vi "Determine E-Series Level_2.vi"(3 "Number of Bands":u8=4 min=3 max=6 step=1, 5 "Tolerance (%)":dbl) -> (1 "E-Series Level":T1)   [LabVIEW 2018]
doc: "Determines the <b>E-Series Level</b> of a resistor based on its <b>Number of Bands</b> and <b>Tolerance (%)</b>.\n\nThe E-Series Level is an internal classification used by the application to determine which E-Series data must be evaluated for the resistor.\n\nThe classification is defined as follows:\n\nE-SERIES LEVEL CLASSIFICATION\n\nBasic : E3, E6 | ±20 % | 3 bands\nLower : E12, E24 | ±10 %, ±5 %, ±2 % | 4 bands\nMiddle : E48 | ±2 % | 5 bands\nHigher : E96 | ±1 % | 5 or 6 bands\nHighest : E192 | ±0.5 %, ±0.25 %, ±0.1 % | 5 or 6 bands\n\nThe resulting <b>E-Series Level</b> identifies the group of E-Series values applicable to the resistor.\n\nThe VI returns the corresponding E-Series Level and provides individual Boolean indicators for Basic, Lower, Middle, Higher, and Highest."
uses:
  E-Series Level--enum.ctl
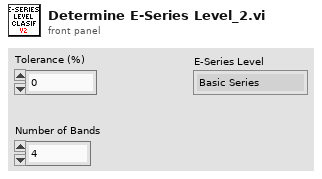
[diagram p1: front panel]
types:
  T1 = typedef "E-Series Level--enum.ctl" = enum16{"Basic Series", "Lower Series", "Middle Series", "Higher Series", "Highest Series"}
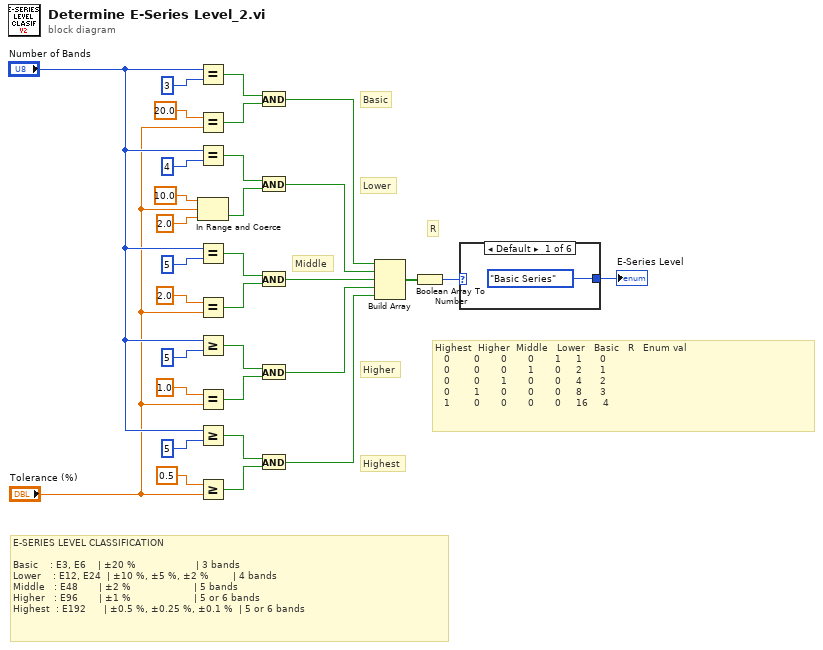
[diagram p0: block diagram]
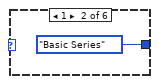
[diagram p2: hidden frame]
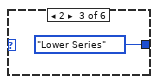
[diagram p3: hidden frame]
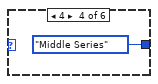
[diagram p4: hidden frame]
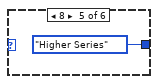
[diagram p5: hidden frame]
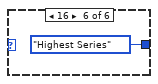
[diagram p6: hidden frame]
diagram:
  # "Middle"
  # "Highest"
  # "Higher"
  # "Lower"
  # "Basic"
  # "R"
  # "Highest  Higher  Middle   Lower   Basic   R   Enum val\n   0        0       0       0       1     1      0\n   0        0       0       1       0     2      1\n   0        0       1       0       0     4      2\n   0        1       0       0       0     8      3\n   1        0       0       0       0     16     4"
  # "E-SERIES LEVEL CLASSIFICATION\n\nBasic    : E3, E6    | ±20 %                    | 3 bands\nLower    : E12, E24  | ±10 %, ±5 %, ±2 %        | 4 bands\nMiddle   : E48       | ±2 %                     | 5 bands\nHigher   : E96       | ±1 %                     | 5 or 6 bands\nHighest  : E192      | ±0.5 %, ±0.25 %, ±0.1 %  | 5 or 6 bands"
  n1 = Equal?(x="Number of Bands", y=u8 3) -> (x = y?=w9:bool)
  n2 = Equal?(x=20.0, y="Tolerance (%)") -> (x = y?=w10:bool)
  n3 = Equal?(x="Number of Bands", y=u8 4) -> (x = y?=w26:bool)
  n4 = In Range and Coerce(upper limit=10.0 ("x"), x="Tolerance (%)", lower limit=2.0) -> (In Range?=w27:bool)  [unwired: 1 out]
  n5 = Equal?(x="Number of Bands", y=u8 5) -> (x = y?=w23:bool)
  n6 = Equal?(x=2.0, y="Tolerance (%)") -> (x = y?=w22:bool)
  n7 = Greater Or Equal?(x="Number of Bands", y=u8 5) -> (x >= y?=w19:bool)
  n8 = Equal?(x=1.0, y="Tolerance (%)") -> (x = y?=w18:bool)
  n9 = Greater Or Equal?(x="Number of Bands", y=u8 5) -> (x >= y?=w14:bool)
  n10 = Greater Or Equal?(x=0.5, y="Tolerance (%)") -> (x >= y?=w13:bool)
  n11 = And(x=w9, y=w10) -> (x .and. y?=w8:bool)
  n12 = And(x=w26, y=w27) -> (x .and. y?=w7:bool)
  n13 = And(x=w23, y=w22) -> (x .and. y?=w6:bool)
  n14 = And(x=w19, y=w18) -> (x .and. y?=w5:bool)
  n15 = And(x=w14, y=w13) -> (x .and. y?=w4:bool)
  n16 = Build Array(w8, w7, w6, w5, w4) -> (w3:bool[])
  n17 = Boolean Array To Number(Boolean array=w3) -> (number=w1:u32)
  n18 = case shown="Default" w1 {
    tunnel: [E-Series_Level--enum."Basic Series" ("E-Series Level") E-Series_Level--enum."Basic Series" ("E-Series Level") E-Series_Level--enum."Lower Series" ("E-Series Level") E-Series_Level--enum."Middle Series" ("E-Series Level") E-Series_Level--enum."Higher Series" ("E-Series Level") E-Series_Level--enum."Highest Series" ("E-Series Level")] -> w2
    frame Default {
    }
    frame 1 {
    }
    frame 2 {
    }
    frame 4 {
    }
    frame 8 {
    }
    frame 16 {
    }
  }
  "E-Series Level" <- w2
